vi "SetObjectConfiguration.vi"(8 "ErrorIn":errorcluster, 9 "DataIn":variant, 10 "Label":string, 11 "ReferenceIn":refnum<class "AppConfigJSON.lvclass">) -> (0 "ErrorOut":errorcluster, 3 "ReferenceOut":refnum<class "AppConfigJSON.lvclass">)   [LabVIEW 2021, in "AppConfigJSON.lvclass"]
uses:
  AppConfigJSON.lvclass
  <vilib>/JDP Science/JSONtext/Config Files/Config File.lvclass/Config File.ctl
  245458c7-ed99-4372-82f3-b56a520705fd.vi
  <vilib>/JDP Science/JSONtext/Variant to JSON Text.vi
  <vilib>/JDP Science/JSONtext/Config Files/Write Config to File.vi
  <vilib>/JDP Science/JSONtext/LVClass Serializer/JSONtext LVClass Serializer.lvclass
  <vilib>/JDP Science/JSONtext/Config Files/Config File.lvclass
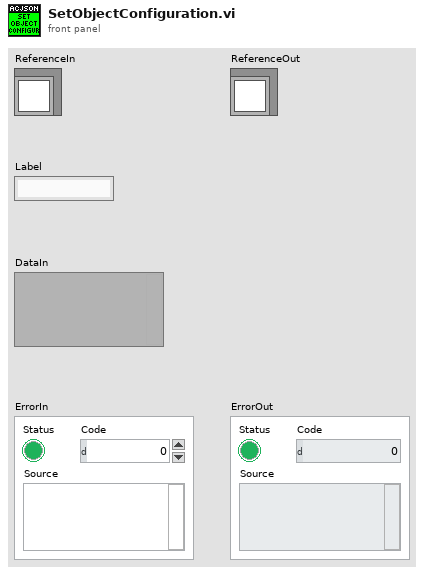
[diagram p1: front panel]
types:
  T1 = typedef "AppConfigJSON.lvclass/ObjectAttributes.ctl" = cluster{"Name":string, "ConfigFilePath":path, "Objects":T2[], "ApplicationBasePath":path, "ObjectName":string}
  T2 = typedef "IApplicationConfiguration.lvclass/ObjectDataDetails.ctl" = cluster{"ObjectName":string, "ObjectType":string, "Interfaces":T3[]}
  T3 = typedef "IApplicationConfiguration.lvclass/ObjectData.ctl" = cluster{"Label":string, "ObjectName":string, "Type":string}
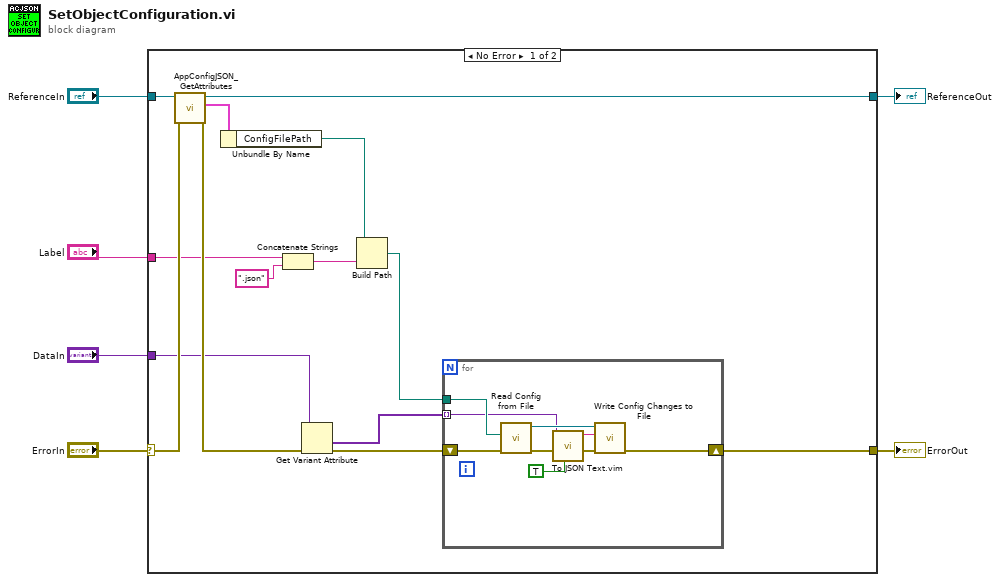
[diagram p0: block diagram]
diagram:
  n1 = case shown="No Error" "ErrorIn" {
    selector: "ErrorIn" -> [w19 w30]
    tunnel: [w17 w30] -> w5
    tunnel: [w14 w29] -> w3
    tunnel: "ReferenceIn" -> [w15 w29]
    tunnel: "Label" -> [w11 _]
    tunnel: "DataIn" -> [w13 _]
    frame No Error {
      n2 = call "AppConfigJSON_GetAttributes.vi"("ErrorIn"=w19, "ReferenceIn"=w15) -> ("ErrorOut"=w18:errorcluster, "Data"=w16:T1, "ReferenceOut"=w14:refnum<class "AppConfigJSON.lvclass">)  [unwired: 6 in, 1 out]
      n3 = Unbundle By Name(w16) -> ("ConfigFilePath"=w12:path)
      n4 = Concatenate Strings(w11, ".json" ("string")) -> (w9:string)
      n5 = Get Variant Attribute(Variant=w13, error in=w18) -> (values=w7:variant[])  [unwired: 2 in, 3 out]
      n6 = Build Path(base path=w12, name or relative path=w9) -> (appended path=w10:path)
      n7 = for {
        tunnel: w10 -> [w22]
        tunnel: w7 -> [w21] mode=indexing
        shift-right: [w25] -> w17
        shift-left: w18 -> [w26]
        n8 = call <vilib>:"Read Config from File.vi"("error in (no error)"=w26, "config file path"=w22) -> ("error out"=w28:errorcluster, "Config File"=w24:refnum<class "Config File.lvclass">)  [unwired: 6 in, 2 out]
        n9 = call "To JSON Text.vim"("Pretty Print?"=TRUE, "error in (no error)"=w28, "Anything"=w21) -> ("error out"=w27:errorcluster, "<JSON>"=w23:string)  [unwired: 7 in]
        n10 = call <vilib>:"Write Config Changes to File.vi"("error in (no error)"=w27, "New Config"=w23, "Config File in"=w24) -> ("error out"=w25:errorcluster)  [unwired: 5 in, 3 out]
      }
    }
    frame Error {
    }
  }
  "ErrorOut" <- w5
  "ReferenceOut" <- w3
